vi "Parse String.vi"(8 "error in (no error)":errorcluster, 11 "JSON Parser in":refnum<class "JSON Parser.lvclass">) -> (0 "error out":errorcluster, 2 "Parsed String":string, 3 "JSON Parser out":refnum<class "JSON Parser.lvclass">)   [LabVIEW 2013, in "JKI JSON Serialization.lvlib" / "JSON Parser.lvclass"]
uses:
  JSON Parser.lvclass
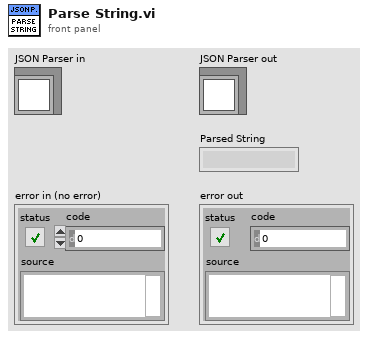
[diagram p1: front panel]
types:
  T1 = typedef "JKI JSON Serialization.lvlib/JSON Lexer.lvclass/JSON Token Type.ctl" = enum32{"unknown", "comma", "end-label", "begin-object", "end-object", "begin-array", "end-array", "quoted-string", "boolean", "exponential-number", "decimal-number", "integer-number", "special-number", "null", "symbol", "whitespace", "EOF"}
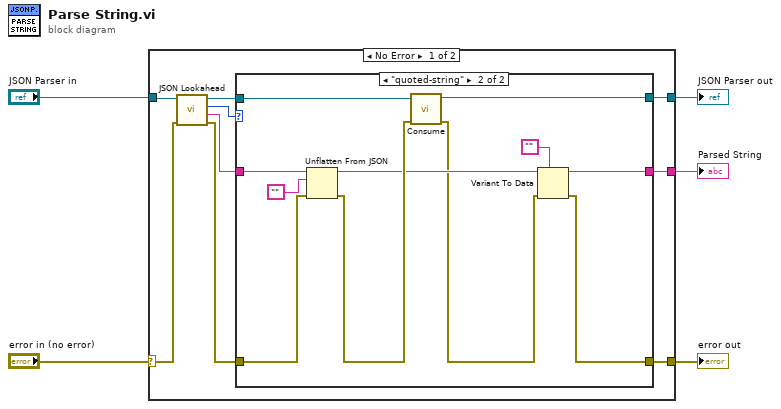
[diagram p0: block diagram]
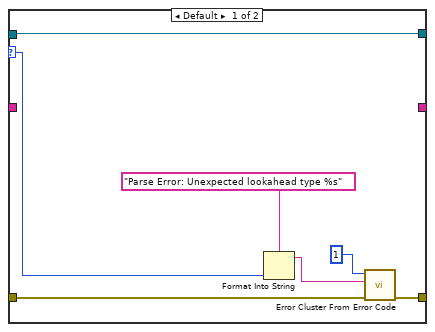
[diagram p2: hidden frame]
diagram:
  n1 = case shown="No Error" "error in (no error)" {
    selector: "error in (no error)" -> [w10 w33]
    tunnel: "JSON Parser in" -> [w11 w34]
    tunnel: [w14 w34] -> w2
    tunnel: [w12 w33] -> w3
    tunnel: [w13 _] -> w4
    frame No Error {
      n2 = call "JSON Lookahead.vi"("error in (no error)"=w10, "Alpaca CLI Parser in"=w11) -> ("error out"=w9:errorcluster, "Lookahead Value"=w6:string, "Lookahead Type"=w7:T1, "Alpaca CLI Parser out"=w8:refnum<class "JSON Parser.lvclass">)  [unwired: 6 in]
      n3 = case shown="\"quoted-string\"" w7 {
        selector: w7 -> [w17 _]
        tunnel: [w21 w32] -> w14
        tunnel: w6 -> [_ w31]
        tunnel: [_ w26] -> w13
        tunnel: [w15 w24] -> w12
        tunnel: w9 -> [w16 w23]
        tunnel: w8 -> [w21 w22]
        frame Default {
          n4 = Format Into String(format string="Parse Error: Unexpected lookahead type %s" ("error message (\"\")"), w17) -> (resulting string=w18:string)  [unwired: 2 in, 1 out]
          n5 = call <vilib>:"Error Cluster From Error Code.vi"("error in (no error)"=w16, "error message (\"\")"=w18, "error code (0)"=1) -> ("error out"=w15:errorcluster)  [unwired: 6 in]
        }
        frame "quoted-string" {
          n6 = Unflatten From JSON(JSON string=w31, type and defaults="", error in (no error)=w23) -> (value=w27:string, error out=w29:errorcluster)  [unwired: 4 in]
          n7 = call-dynamic "Consume.vi"("error in (no error)"=w29, "Alpaca Parser in"=w22) -> ("error out"=w25:errorcluster, "Alpaca Parser out"=w32:refnum<class "JSON Parser.lvclass">)  [unwired: 8 in]
          n8 = Variant To Data(error in=w25, type="", Variant=w27) -> (data=w26:string, error out=w24:errorcluster)
        }
      }
    }
    frame Error {
    }
  }
  "Parsed String" <- w4
  "error out" <- w3
  "JSON Parser out" <- w2
